vi "getAttributeTreeUnitTooltip.vi"(0 "HGF_IMAQDevice":refnum<class "HGF_IMAQDevice.lvclass">, 1 "Tree Control In":refnum<vi>, 2 "Force update?":bool, 3 "Tab Control Ref In":T1, 5 "error in (no error)":errorcluster) -> (14 "dup HGF_IMAQDevice":refnum<class "HGF_IMAQDevice.lvclass">, 15 "Tree Control Out":refnum<vi>, 16 "Units":string, 17 "Tooltip":string, 19 "error out":errorcluster)   [LabVIEW 2014, in "HGF_IMAQ.lvlib" / "HGF_IMAQDevice.lvclass"]
doc: "This is the override VI to read cameras attribute unit and tooltip."
uses:
  HGF_IMAQDevice.lvclass
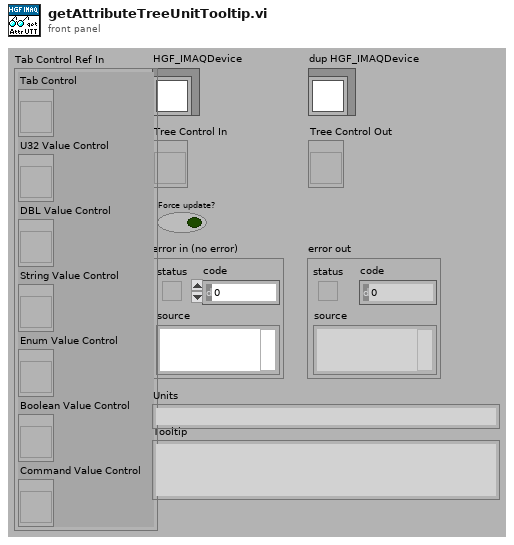
[diagram p1: front panel]
types:
  T1 = cluster{"Tab Control":refnum<vi>, "U32 Value Control":refnum<vi>, "DBL Value Control":refnum<vi>, "String Value Control":refnum<vi>, "Enum Value Control":refnum<vi>, "Boolean Value Control":refnum<vi>, "Command Value Control":refnum<vi>}
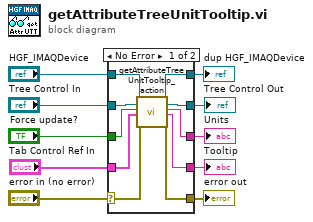
[diagram p0: block diagram]
diagram:
  n1 = case shown="No Error" "error in (no error)" {
    selector: "error in (no error)" -> [w20 w21]
    tunnel: [w19 w21] -> w9
    tunnel: [w16 w22] -> w7
    tunnel: "HGF_IMAQDevice" -> [w17 w22]
    tunnel: "Tree Control In" -> [w18 _]
    tunnel: [w15 _] -> w5
    tunnel: "Force update?" -> [w14 _]
    tunnel: "Tab Control Ref In" -> [w13 _]
    tunnel: [w12 _] -> w2
    tunnel: [w11 _] -> w1
    frame No Error {
      n2 = call-dynamic "getAttributeTreeUnitTooltip_action.vi"("HGF_IMAQDevice"=w17, "Tree Control In"=w18, "Force update?"=w14, "Tab Control Ref In"=w13, "error in (no error)"=w20) -> ("dup HGF_IMAQDevice"=w16:refnum<class "HGF_IMAQDevice.lvclass">, "Tree Control Out"=w15:refnum<vi>, "Units"=w12:string, "Tooltip"=w11:string, "error out"=w19:errorcluster)  [unwired: 10 in]
    }
    frame Error {
    }
  }
  "error out" <- w9
  "dup HGF_IMAQDevice" <- w7
  "Tree Control Out" <- w5
  "Tooltip" <- w1
  "Units" <- w2
